vi "chart series set marker size.vi"(8 "error in (no error)":errorcluster, 10 "size":u8, 11 "series":u32) -> (0 "error out":errorcluster)   [LabVIEW 8.6]
doc: "void chart_series_set_marker_size(lxw_chart_series series, uint8_t size);"
uses:
  pending_lvxlsxwriter/xlsxwriter.dll
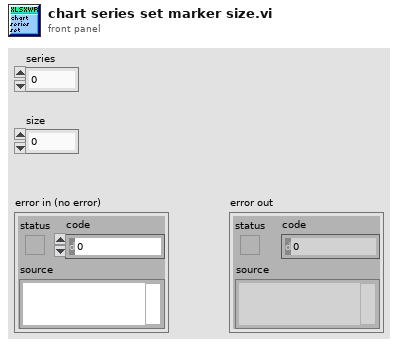
[diagram p1: front panel]
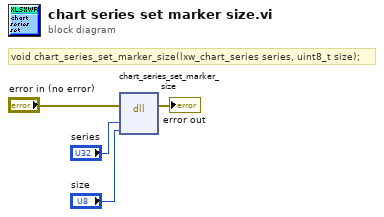
[diagram p0: block diagram]
diagram:
  # "void chart_series_set_marker_size(lxw_chart_series series, uint8_t size);"
  n1 = dll-call lib="C:/Users/WDAGUtilityAccount/Desktop/pending_lvxlsxwriter/xlsxwriter.*" fn="chart_series_set_marker_size"(error in="error in (no error)", "series"="series", "size"="size") -> (error out=→"error out":errorcluster)  [unwired: 5 in, 1 out]
